vi "TimedBytesAtSerialPort.vi"(9 "Time-out (5 Secs)":dbl=5.0 format="%.2f", 10 "Byte count":u32=1, 11 "Serial port (0)":i32) -> (1 "Time-out?":bool, 2 "Bytes count":u32, 3 "String read":string)   [LabVIEW 2010]
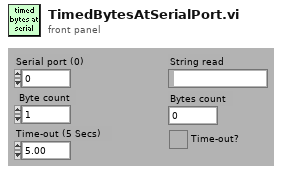
[diagram p1: front panel]
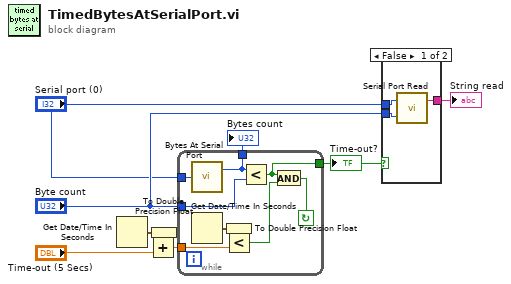
[diagram p0: block diagram]
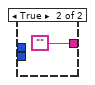
[diagram p2: hidden frame]
diagram:
  n1 = Get Date/Time In Seconds() -> (seconds since 1Jan1904=w1:timestamp)
  n2 = To Double Precision Float(number=w1) -> (double precision float=w9:dbl)
  n3 = Add(x=w9, y="Time-out (5 Secs)") -> (x+y=w8:dbl)
  n4 = while {
    tunnel: [w11] -> w2
    tunnel: "Byte count" -> [w13]
    tunnel: [w14] -> w6
    tunnel: w8 -> [w18]
    tunnel: "Serial port (0)" -> [w16]
    stop <- w15 continue-if-true
    n5 = call <vilib>:"Bytes At Serial Port.vi"("port number"=w16) -> ("byte count"=w14:u32)  [unwired: 1 out]
    n6 = Get Date/Time In Seconds() -> (seconds since 1Jan1904=w10:timestamp)
    n7 = To Double Precision Float(number=w10) -> (double precision float=w17:dbl)
    n8 = Less?(x=w17, y=w18) -> (x < y?=w12:bool)
    n9 = Less?(x=w14, y=w13) -> (x < y?=w11:bool)
    n10 = And(x=w11, y=w12) -> (x .and. y?=w15:bool)
  }
  "Time-out?" <- w2
  "Bytes count" <- w6
  n11 = case shown="False" w2 {
    tunnel: "Byte count" -> [w20 _]
    tunnel: "Serial port (0)" -> [w21 _]
    tunnel: [w19 ""] -> w3
    frame False {
      n12 = call <vilib>:"Serial Port Read.vi"("requested byte count"=w20, "port number"=w21) -> ("string read"=w19:string)  [unwired: 1 out]
    }
    frame True {
    }
  }
  "String read" <- w3
